vi "Read Connection Information.vi"(11 "Websocket Client Handler in":refnum<class "Websocket Client Handler.lvclass">) -> (3 "Websocket Client Handler out":refnum<class "Websocket Client Handler.lvclass">, 4 "Remote Address":string, 6 "Connection ID":refnum<k5>)   [LabVIEW 2016, in "Stream Mediator.lvlib" / "Websocket Client Handler.lvclass"]
doc: "--\nCopyright © 2017 Composed SystemsI All rights reserved.\n\nAuthor: Jon McBee <jon.mcbee@composed.io>\n\nThis library is provided \"AS IS\" ,WITHOUT WARRANTIES OR\nCONDITIONS OF ANY KIND, either express or implied.\n\nComposed Systems -- composed.io\n\nStream 0.0.1.1\nJon McBee - Composed Systems\nCopyright (c) 2017, Composed Systems"
uses:
  <userlib>/Composed Systems/Stream/Mediator/Classes/Websocket Client Handler Actor/Websocket Client Handler/Websocket Client Handler.lvclass
  <userlib>/Composed Systems/Stream/Mediator/Classes/Websocket Client Handler Actor/Websocket Client Handler/Websocket Client Handler.lvclass/Websocket Client Handler.ctl
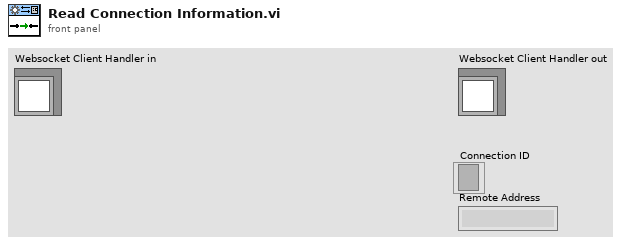
[diagram p1: front panel]
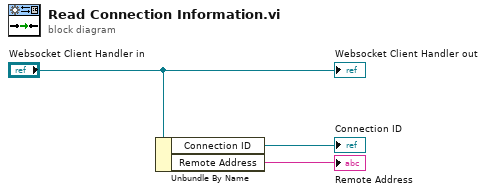
[diagram p0: block diagram]
diagram:
  n1 = Unbundle By Name("Websocket Client Handler in") -> ("Connection ID"=→"Connection ID":refnum<k5>, "Remote Address"=→"Remote Address":string)
  "Websocket Client Handler out" <- "Websocket Client Handler in"
